vi "Send Email.vi"() -> ()   [LabVIEW 2014]
uses:
  <vilib>/smtpClient/Set Message Text.vi
  <vilib>/smtpClient/LabVIEWSMTPClient.lvlib
panel:
  in  "username":string
  in  "server address":string
  in  "attachments":path[](array[path])
  in  "plain text message":string
  in  "subject":string
  in  "password":string
  in  "from":string
  in  "to":string[](array[string])
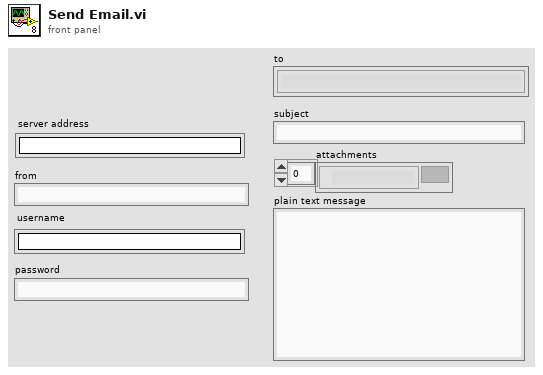
[diagram p1: front panel]
types:
  T1 = typedef "LabVIEWSMTPClient.lvlib/SmtpClientHandle.ctl" = refnum<k1>
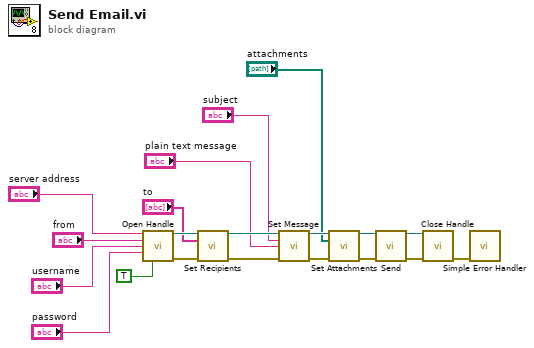
[diagram p0: block diagram]
diagram:
  n1 = call <vilib>:"Open Handle.vi"("server address"="server address", "from"="from", "username"="username", "password"="password", "use TLS (false)"=TRUE) -> ("handle out"=w18:T1, "error out"=w16:errorcluster)  [unwired: 9 in]
  n2 = call <vilib>:"Set Recipients.vi"("handle in"=w18, "to"="to", "error in (no error)"=w16) -> ("handle out"=w15:T1, "error out"=w12:errorcluster)  [unwired: 11 in]
  n3 = call-poly <vilib>:"Set Message.vi"("handle in"=w15, "subject"="subject", "plain text message"="plain text message", "error in (no error)"=w12) -> ("handle out"=w6:T1, "error out"=w7:errorcluster)  [unwired: 10 in]
  n4 = call <vilib>:"Set Attachments.vi"("handle in"=w6, "attachments"="attachments", "error in (no error)"=w7) -> ("handle out"=w5:T1, "error out"=w4:errorcluster)  [unwired: 11 in]
  n5 = call <vilib>:"Send.vi"("handle in"=w5, "error in (no error)"=w4) -> ("handle out"=w11:T1, "error out"=w10:errorcluster)  [unwired: 11 in, 1 out]
  n6 = call <vilib>:"Close Handle.vi"("handle in"=w11, "error in (no error)"=w10) -> ("error out"=w9:errorcluster)  [unwired: 12 in, 1 out]
  n7 = call <vilib>:"Simple Error Handler.vi"("error in (no error)"=w9) -> ()  [unwired: 4 in, 5 out]
